vi "fgv_erp42mini-data.vi"(7 "cmd":enum16{"ini", "write", "read"}(ring), 8 "error in":errorcluster, 11 "erp_read-data":string) -> (0 "error out":errorcluster, 3 "output cluster":T1)   [LabVIEW 2019]
panel:
  out "steer-cal":dbl
  out "Waveform Chart":u32(graph)
  out "dt":u32
  out "Encoder_Reset":u8
  out "GM_Lidar_L":u16
  out "GM_Lidar_R":u16
  out "Encoder":i32
  out "Brake":i16
  out "Steer":i16
  out "Speed-r":u16
  out "Direction":u8
  out "M/A":u8
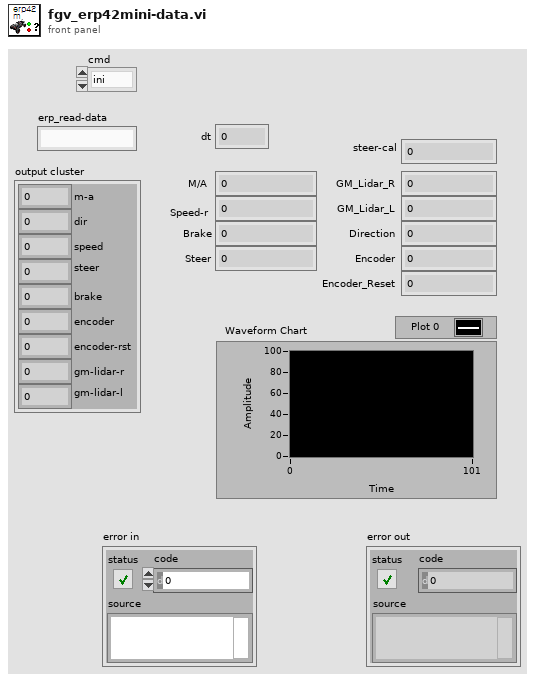
[diagram p1: front panel]
types:
  T1 = cluster{"m-a":u8, "dir":u8, "speed":u16, "steer":i16, "brake":i16, "encoder":i32, "encoder-rst":u8, "gm-lidar-r":u16, "gm-lidar-l":u16}
  T2 = cluster{"Numeric":u8, "Numeric":u8, u16, i16, i16, i32, "Numeric":u8, u16, u16}
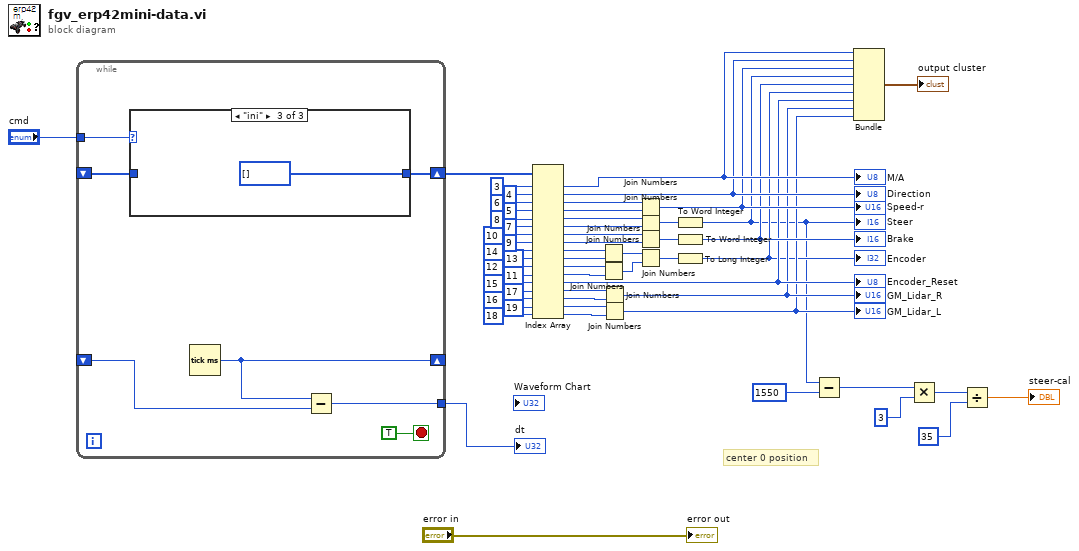
[diagram p0: block diagram]
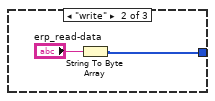
[diagram p3: hidden frame]
diagram:
  # "center 0 position"
  n1 = while {
    tunnel: "cmd" -> [w62]
    shift-right: [w61] -> w19
    shift-left: _ -> [w60]
    shift-right: [w57] -> _
    shift-left: _ -> [w59]
    tunnel: [w58] -> w2
    stop <- TRUE stop-if-true
    n2 = case shown="\"ini\"" w62 {
      tunnel: [w64 w65 u8[] [] ("erp-data-in")] -> w61
      tunnel: w60 -> [w64 _ _]
      frame "read", Default {
      }
      frame "write" {
        n3 = String To Byte Array(string="erp_read-data") -> (unsigned byte array=w65:u8[])
      }
      frame "ini" {
      }
    }
    n4 = Tick Count (ms)() -> (millisecond timer value=w57:u32)
    n5 = Subtract(x=w57, y=w59) -> (x-y=w58:u32)
  }
  "dt" <- w2
  n6 = Index Array(array=w19, index #1=3, index #2=4, index #3=6, index #4=5, index #5=8, index #6=7, index #7=10, index #8=9, index #9=14, index #10=13, index #11=12, index #12=11, index #13=15, index #14=17, index #15=16, index #16=19, index #17=18) -> (element #1=w18:u8, element #2=w17:u8, element #3=w39:u8, element #4=w38:u8, element #5=w37:u8, element #6=w36:u8, element #7=w35:u8, element #8=w34:u8, element #9=w32:u8, element #10=w33:u8, element #11=w31:u8, element #12=w30:u8, element #13=w14:u8, element #14=w21:u8, element #15=w20:u8, element #16=w23:u8, element #17=w22:u8)
  "M/A" <- w18
  "Direction" <- w17
  "Encoder_Reset" <- w14
  n7 = Join Numbers(hi=w32, lo=w33) -> ((hi.lo)=w28:u16)
  n8 = Join Numbers(hi=w31, lo=w30) -> ((hi.lo)=w29:u16)
  n9 = Join Numbers(hi=w21, lo=w20) -> ((hi.lo)=w13:u16)
  "GM_Lidar_R" <- w13
  n10 = Join Numbers(hi=w23, lo=w22) -> ((hi.lo)=w11:u16)
  "GM_Lidar_L" <- w11
  n11 = Join Numbers(hi=w39, lo=w38) -> ((hi.lo)=w16:u16)
  "Speed-r" <- w16
  n12 = Join Numbers(hi=w37, lo=w36) -> ((hi.lo)=w27:u16)
  n13 = Join Numbers(hi=w35, lo=w34) -> ((hi.lo)=w26:u16)
  n14 = Join Numbers(hi=w28, lo=w29) -> ((hi.lo)=w25:u32)
  n15 = To Word Integer(number=w27) -> (16bit integer=w9:i16)
  "Steer" <- w9
  n16 = To Word Integer(number=w26) -> (16bit integer=w15:i16)
  "Brake" <- w15
  n17 = To Long Integer(number=w25) -> (32bit integer=w10:i32)
  "Encoder" <- w10
  n18 = Subtract(x=w9, y=i16 1550) -> (x-y=w7:i16)
  n19 = Bundle("Numeric"=w18, "Numeric"=w17, w16, w9, w15, w10, "Numeric"=w14, w13, w11) -> (→"output cluster":T2)  [unwired: 1 in]
  n20 = Multiply(x=w7, y=i16 3) -> (x*y=w5:i16)
  n21 = Divide(x=w5, y=i16 35) -> (x/y=→"steer-cal":dbl)
  "error out" <- "error in"
